vi "State_Machine.vi"(8 "error in (no error)":errorcluster caption="entrée d'erreur (pas d'erreur)", 11 "Delay en entrée":refnum<class "Delay.lvclass">) -> (0 "error out":errorcluster caption="sortie d'erreur", 2 "Json_String":string, 3 "Delay en sortie":refnum<class "Delay.lvclass">)   [LabVIEW 2020, in "Library Test.lvlib" / "Delay.lvclass"]
uses:
  Delay.lvclass
  C:/Users/ngarcin/OneDrive - Altyor/Standard TB/Class/Test/Test (Default)/Test (Default).lvclass
  JSON API/JSON Value/Set from JSON string.vi
  JSON API/JSON Value/JSON Value.lvclass
  Delay.lvclass/Delay.ctl
  Commun VI/Library Commun.lvlib
  JSON API/Variant JSON/Variant JSON.lvlib
  JSON API/Get Polymorphic/JSON GetSet.lvlib
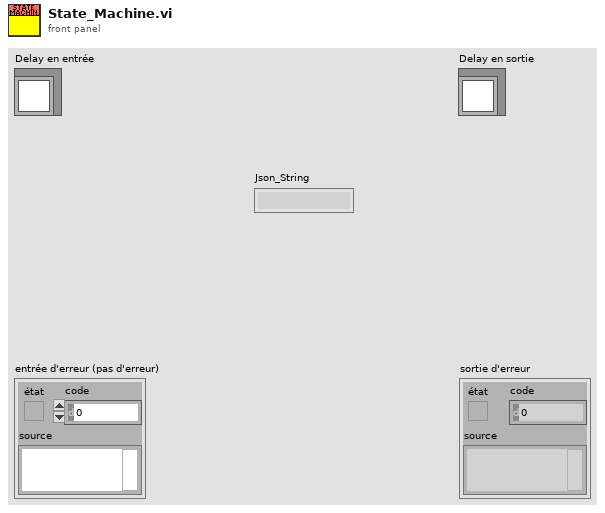
[diagram p1: front panel]
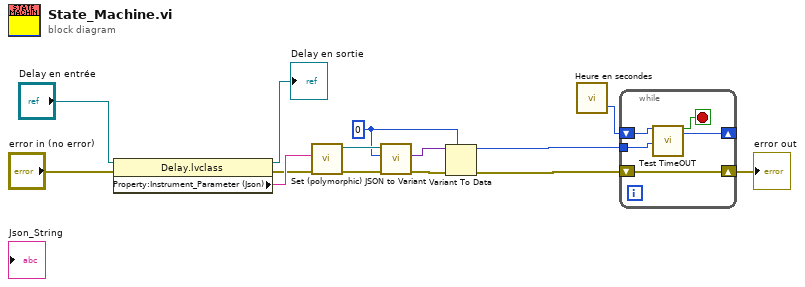
[diagram p0: block diagram]
diagram:
  w8 = u32 0 ("Channel")
  n1 = property class="Delay.lvclass"(reference="Delay en entrée", error in="error in (no error)") -> (reference out=→"Delay en sortie":refnum<class "Delay.lvclass">, error out=w2:errorcluster, "Property:Instrument_Parameter (Json)"=w7:string)
  n2 = call-poly "Set (polymorphic).vi"("error in (no error)"=w2, "JSON stream"=w7) -> ("error out"=w10:errorcluster, "JSON Value out"=w12:refnum<class "JSON Value.lvclass">)  [unwired: 7 in, 1 out]
  n3 = call "JSON to Variant.vi"("error in (no error)"=w10, "Variant (Data Type)"=w8, "JSON Value"=w12) -> ("error out"=w11:errorcluster, "Variant out"=w9:variant)  [unwired: 7 in]
  n4 = Variant To Data(error in=w11, type=w8, Variant=w9) -> (data=w1:u32, error out=w5:errorcluster)
  n5 = call "Heure en secondes.vi"() -> ("Heure en milisecondes"=w14:u32)  [unwired: 2 in, 1 out]
  n6 = while {
    shift-right: [w18] -> _
    shift-left: w14 -> [w19]
    shift-right: [w17] -> w3
    shift-left: w5 -> [w17]
    tunnel: w1 -> [w16]
    stop <- w15 stop-if-true
    n7 = call "Test TimeOUT.vi"("OLD Time"=w19, "TimeOut ms"=w16) -> ("Timeout ?"=w15:bool, "NEW Time"=w18:u32)  [unwired: 13 in, 3 out]
  }
  "error out" <- w3
